vi "Moz Test.vi"() -> ()   [LabVIEW 2017]
panel:
  in  "String":string
  in  "MozillaBrowser":refnum<k7>(container)
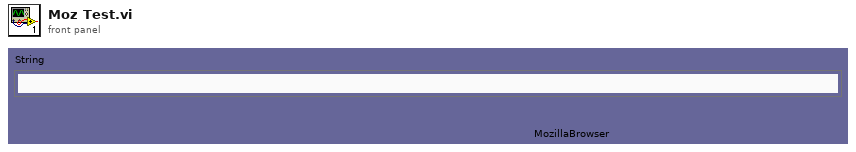
[diagram p1: front panel]
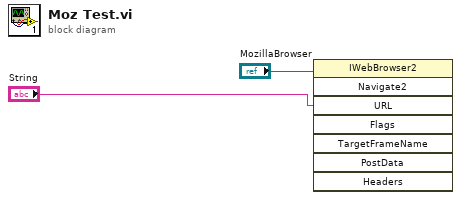
[diagram p0: block diagram]
diagram:
  n1 = invoke class="IWebBrowser2" method="Navigate2"(reference="MozillaBrowser", "URL"="String") -> ()  [unwired: 6 in, 8 out]
